vi "Strip Actor Name.vi"(10 "Characters From End To Strip":i32=19, 11 "Actor Name in":string) -> (3 "Actor Name out":string)   [LabVIEW 2015, in "Debugger.lvclass"]
uses:
  Debugger.lvclass
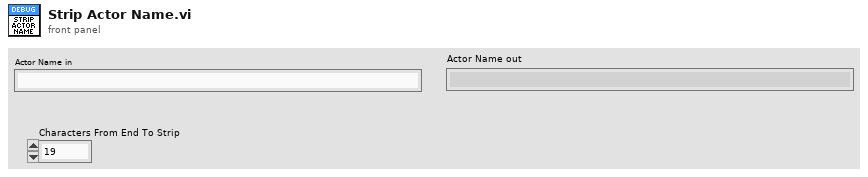
[diagram p1: front panel]
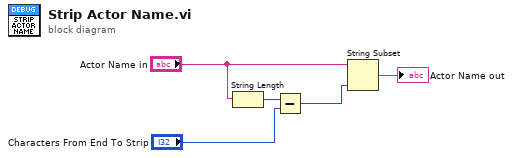
[diagram p0: block diagram]
diagram:
  n1 = String Length(string="Actor Name in") -> (length=w5:i32)
  n2 = Subtract(x=w5, y="Characters From End To Strip") -> (x-y=w4:i32)
  n3 = String Subset(string="Actor Name in", length (rest)=w4) -> (substring=→"Actor Name out":string)  [unwired: 1 in]
